vi "Register for Sequence State Change Event.vi"(8 "error in (no error)":errorcluster, 10 "Sequence Names":string[](array[string]), 11 "Session Ref in":T2) -> (0 "error out":errorcluster, 1 "Event Registration Refnum":refnum<event-registration>, 2 "Sequence Names out":string[](array[string]), 3 "Session Ref out":T2, 5 "Sequence State Change Event Ref":T1)   [LabVIEW 2020, in "NI_VS Sequence Execution Interface.lvlib"]
doc: "Registers for a state change event for a set of sequences you specify. A state change event is triggered any time a sequence changes execution state. This VI returns a registered user event reference and information about the event."
uses:
  <vilib>/NI VeriStand/Execution/SequenceExecutionInterface/NI_VS Sequence Execution Interface.lvlib
  <vilib>/NI VeriStand/Execution/SequenceExecutionInterface/Stimulus Profile Session Ref.ctl
  NationalInstruments.VeriStand.ClientAPI
  <vilib>/NI VeriStand/Execution/SequenceExecutionInterface/Sequence State Change Event Ref.ctl
  <vilib>/NI VeriStand/Execution/SequenceExecutionInterface/Sequence State Change Event Data.ctl
  <vilib>/NI VeriStand/Execution/SequenceExecutionInterface/Sequence Execution State.ctl
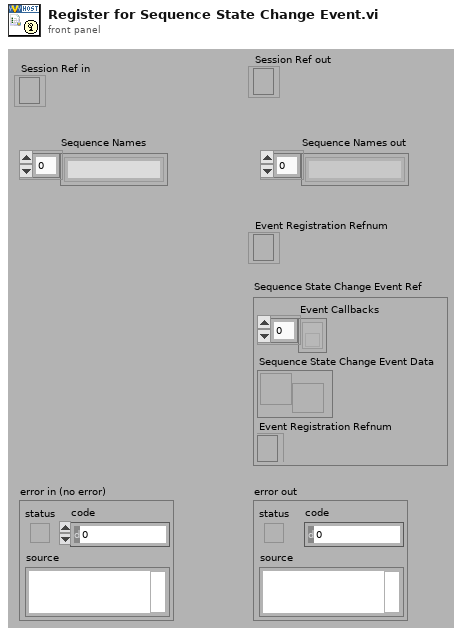
[diagram p1: front panel]
types:
  T1 = typedef "NI_VS Sequence Execution Interface.lvlib/Sequence State Change Event Ref.ctl" = cluster{"Event Callbacks":refnum<k27>[], "Sequence State Change Event Data":refnum<user-event>, "Event Registration Refnum":refnum<event-registration>}
  T2 = typedef "NI_VS Sequence Execution Interface.lvlib/Stimulus Profile Session Ref.ctl" = refnum<k24>
  T3 = typedef "NI_VS Sequence Execution Interface.lvlib/Sequence State Change Event Data.ctl" = cluster{"Sequence Name":string, "State":T4, "Aborted":bool}
  T4 = typedef "NI_VS Sequence Execution Interface.lvlib/Sequence Execution State.ctl" = enum16{"Idle", "Running", "SingleStepping", "Paused", "Stopped"}
  T5 = cluster{refnum<k27>[], "Sequence State Change Event Data":refnum<user-event>, "Event Registration Refnum":refnum<event-registration>}
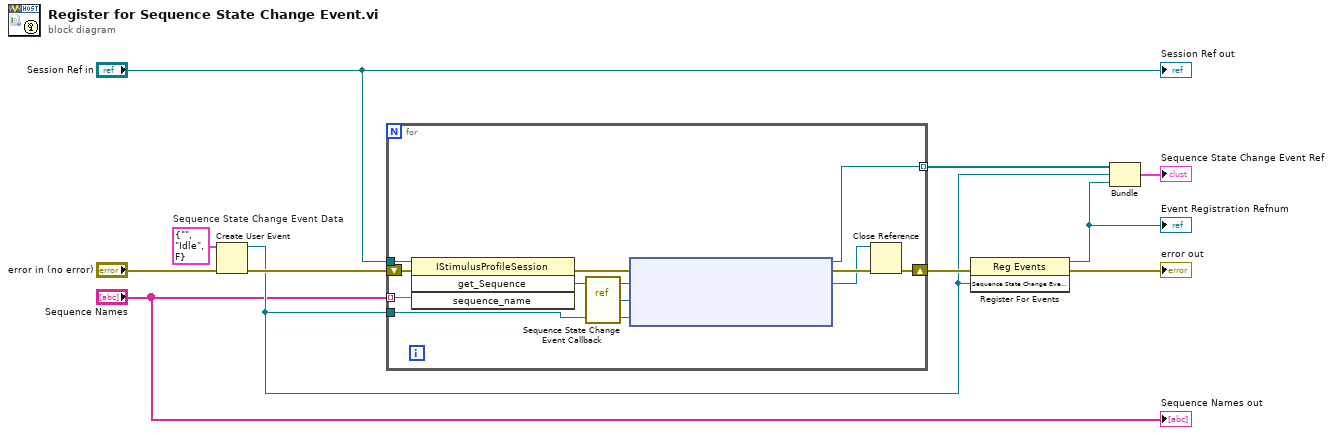
[diagram p0: block diagram]
diagram:
  w4 = T3 {"Sequence Name"="", "State"=enum."Idle", "Aborted"=FALSE}  # Sequence State Change Event Data
  n1 = Create User Event(user event datatype=w4, error in="error in (no error)") -> (user event=w6:refnum<user-event>, error out=w11:errorcluster)
  n2 = for {
    tunnel: [w19] -> w9 mode=indexing
    tunnel: w6 -> [w18]
    tunnel: "Session Ref in" -> [w17]
    shift-right: [w20] -> w10
    shift-left: w11 -> [w21]
    tunnel: "Sequence Names" -> [w12] mode=indexing
    n3 = invoke class="IStimulusProfileSession" method="get_Sequence"(reference=w17, error in=w21, "sequence_name"=w12) -> (error out=w13:errorcluster, "get_Sequence"=w14:refnum<k24>)  [unwired: 1 in, 2 out]
    n4 = vi-ref <vilib>:"Sequence State Change Event Callback.vi"() -> ("vi reference"=w16:refnum<vi>)
    n5 = node(w13, w14, w16, w18) -> (w19:refnum<k27>, w15:errorcluster)  [unwired: 1 in]
    n6 = Close Reference(reference=w14, error in (no error)=w15) -> (error out=w20:errorcluster)
  }
  n7 = register-events(error in=w10, w6) -> (reference out=w7:refnum<event-registration>, error out=→"error out":errorcluster)  [unwired: 1 in]
  "Event Registration Refnum" <- w7
  n8 = Bundle(w9, "Sequence State Change Event Data"=w6, "Event Registration Refnum"=w7) -> (→"Sequence State Change Event Ref":T5)  [unwired: 1 in]
  "Session Ref out" <- "Session Ref in"
  "Sequence Names out" <- "Sequence Names"
